vi "OOK_Demodulation.vi"(9 "trigger level":dbl, 10 "downsampling factor":i32, 11 "input symbol stream":cdb[](array[numeric])) -> (3 "output bit stream":i8[](array[numeric]))   [LabVIEW 2014]
uses:
  <vilib>/Analysis/baseanly.llb/Mean (DBL).vi
  <vilib>/Analysis/NI_AALBase.lvlib
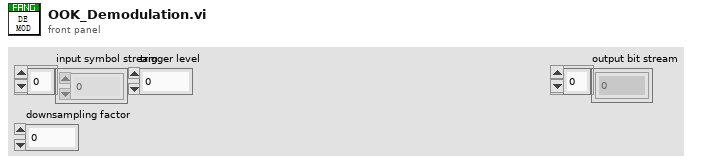
[diagram p1: front panel]
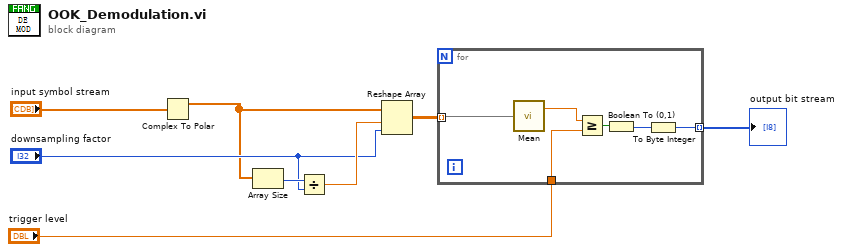
[diagram p0: block diagram]
diagram:
  n1 = Complex To Polar(r * e^(i*theta)="input symbol stream") -> (r=w3:dbl[])  [unwired: 1 out]
  n2 = Array Size(array=w3) -> (size(s)=w8:i32)
  n3 = Divide(x=w8, y="downsampling factor") -> (x/y=w7:dbl)
  n4 = Reshape Array(w3, w7, "downsampling factor") -> (w5:dbl[][])
  n5 = for {
    tunnel: w5 -> [w14] mode=indexing
    tunnel: "trigger level" -> [w12]
    tunnel: [w9] -> w1 mode=indexing
    n6 = call-poly <vilib>:"Mean.vi"("X"=w14) -> ("mean"=w13:dbl)  [unwired: 1 out]
    n7 = Greater Or Equal?(x=w13, y=w12) -> (x >= y?=w11:bool)
    n8 = Boolean To (0,1)(Boolean=w11) -> (0, 1=w10:i16)
    n9 = To Byte Integer(number=w10) -> (8bit integer=w9:i8)
  }
  "output bit stream" <- w1
